vi "f_MGCC_PVFcst_ActualPV.vi"() -> ()   [LabVIEW 2016]
panel:
  in  "ActualPV":dbl[](array[numeric])
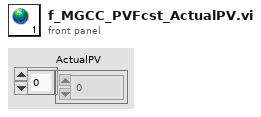
[diagram p1: front panel]
diagram:
